vi "Max Bin Read (single queue) ALTERNATIVE.vi"(0 "FPGA VI Reference In":refnum<k20>) -> (14 "Max Bin":i32, 15 "Max Amp":dbl, 16 "Next Bin":i32, 17 "Next Amp":dbl, 18 "Prev Bin":i32, 19 "Prev Amp":dbl)   [LabVIEW 2014]
uses:
  <vilib>/Utility/error.llb/Error Cluster From Error Code.vi
  <vilib>/rvi/errors/niLvFpgaAdjustHostInterfaceError.vi
  <vilib>/rvi/interface/nirviMethod/nirviMethod.xnode
  <vilib>/FPGAPlugInAG/Dynamic/niLvFpga_ReadFifo_Dynamic.vi
  <vilib>/rvi/errors/niLvFpgaMergeErrorWithErrorCode.vi
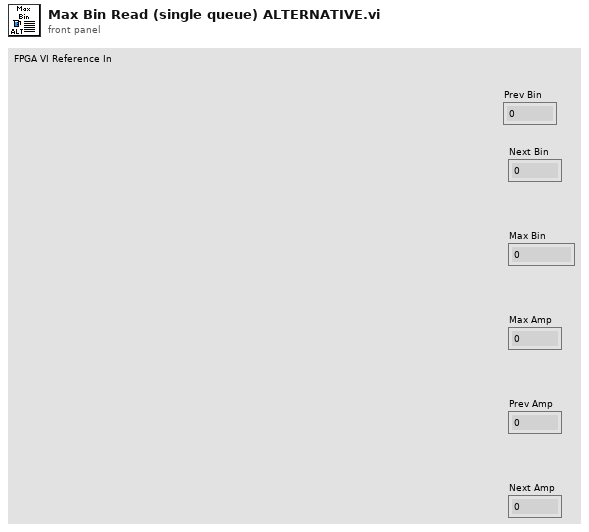
[diagram p1: front panel]
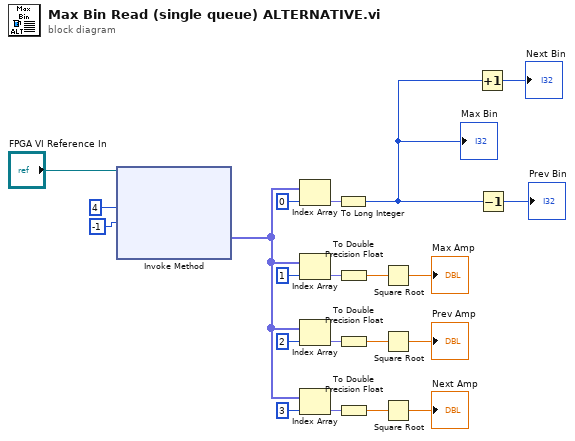
[diagram p0: block diagram]
diagram:
  n1 = xnode "Invoke Method"("FPGA VI Reference In"="FPGA VI Reference In", "Number of Elements"=u32 4, "Timeout (ms)"=-1) -> ("Data"=w3:fxp<+,44,44>[])  [unwired: 1 in, 3 out]
  n2 = Index Array(array=w3, index=0) -> (element=w2:fxp<+,44,44>)
  n3 = Index Array(array=w3, index=1) -> (element=w16:fxp<+,44,44>)
  n4 = Index Array(array=w3, index=2) -> (element=w12:fxp<+,44,44>)
  n5 = Index Array(array=w3, index=3) -> (element=w7:fxp<+,44,44>)
  n6 = To Long Integer(number=w2) -> (32bit integer=w20:i32)
  "Max Bin" <- w20
  n7 = To Double Precision Float(number=w16) -> (double precision float=w15:dbl)
  n8 = To Double Precision Float(number=w12) -> (double precision float=w11:dbl)
  n9 = To Double Precision Float(number=w7) -> (double precision float=w8:dbl)
  n10 = Square Root(x=w15) -> (sqrt(x)=→"Max Amp":dbl)
  n11 = Square Root(x=w11) -> (sqrt(x)=→"Prev Amp":dbl)
  n12 = Square Root(x=w8) -> (sqrt(x)=→"Next Amp":dbl)
  n13 = Increment(x=w20) -> (x+1=→"Next Bin":i32)
  n14 = Decrement(x=w20) -> (x-1=→"Prev Bin":i32)
